vi "Climb_Execute.vi"() -> ()   [LabVIEW 2019]
uses:
  Globals/Climb_Globals.vi
  <vilib>/Rock Robotics/WPI/Solenoid/WPI_SolenoidValue.ctl
panel:
  out "LeadScrew_Throttle":dbl
  out "Joint_Power":dbl
  out "Pin":T1=enum."Forward"
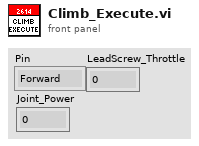
[diagram p1: front panel]
types:
  T1 = typedef "WPI_SolenoidValue.ctl" = enum16{"Off", "On", "Forward", "Reverse"}
  T2 = typedef "Climb_Cluster.ctl" = cluster{"Control_State":enum16{"No-Op", "Extending", "Clamping", "Balancing", "Manual_Control"}, "Extend_Climber?":bool, "Clamp?":bool, "Balance?":bool, "Manual_Control?":bool, "Joint_Throttle":dbl, "LeadScrew_Throttle":dbl}
  T3 = enum16{"No-Op", "Extending", "Clamping", "Balancing", "Manual_Control"}
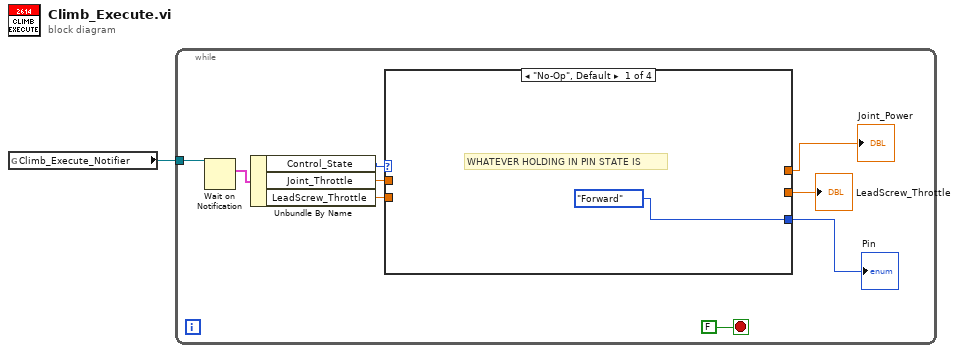
[diagram p0: block diagram]
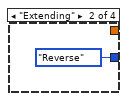
[diagram p2: hidden frame]
diagram:
  n1 = global read "Climb_Globals.vi" "Climb_Execute_Notifier"() -> (w1:refnum<notifier>)
  n2 = while {
    tunnel: w1 -> [w9]
    stop <- FALSE stop-if-true
    n3 = Wait on Notification(notifier=w9) -> (notification=w8:T2)  [unwired: 3 in, 3 out]
    n4 = Unbundle By Name(w8) -> ("Control_State"=w7:T3, "Joint_Throttle"=w5:dbl, "LeadScrew_Throttle"=w3:dbl)
    n5 = case shown="\"No-Op\", Default" w7 {
      tunnel: [WPI_SolenoidValue."Forward" ("Value") WPI_SolenoidValue."Reverse" ("Value") _ _] -> w6
      tunnel: w5 -> [_ _ _ w14]
      tunnel: [_ _ _ w14] -> w4
      tunnel: w3 -> [_ _ w13 _]
      tunnel: [_ _ w13 _] -> w2
      frame "No-Op", Default {
        # "WHATEVER HOLDING IN PIN STATE IS"
      }
      frame "Extending" {
      }
      frame "Clamping" {
        # "fully manual control atm"
      }
      frame "Balancing" {
        # "all manual right now, add in auto-balance"
      }
    }
    "Pin" <- w6
    "Joint_Power" <- w4
    "LeadScrew_Throttle" <- w2
  }
